vi "get_base_directories.vi"() -> (0 "data_base_dir":path=path "F:/data", 1 "stimuli_base_dir":path=path "C:/code/auditory-physiology/stimuli", 2 "protocols_base_dir":path=path "C:/code/auditory-physiology/protocols", 3 "metadata_base_dir":path=path "C:/code/auditory-physiology/metadata")   [LabVIEW 2015]
panel:
  # "Default Directories For metadata, protocol, stimuli, data etc.,"
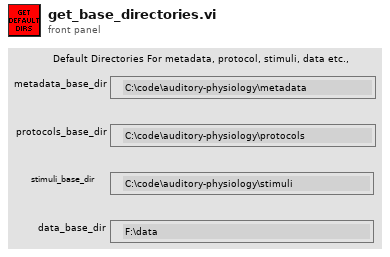
[diagram p1: front panel]
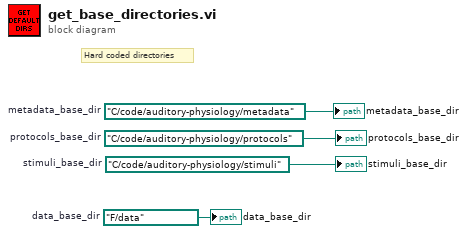
[diagram p0: block diagram]
diagram:
  w1 = path "F:/data"  # data_base_dir
  w3 = path "C:/code/auditory-physiology/protocols"  # protocols_base_dir
  w4 = path "C:/code/auditory-physiology/metadata"  # metadata_base_dir
  w2 = path "C:/code/auditory-physiology/stimuli"  # stimuli_base_dir
  # "Hard coded directories"
  "metadata_base_dir" <- w4
  "protocols_base_dir" <- w3
  "stimuli_base_dir" <- w2
  "data_base_dir" <- w1
